vi "Configure C4209.vi"(8 "error in (no error)":errorcluster, 11 "C4209 PNA":refnum<class "C4209 PNA.lvclass">) -> (0 "error out":errorcluster, 3 "C4209 PNA out":refnum<class "C4209 PNA.lvclass">)   [LabVIEW 2017, in "C4209 PNA.lvclass"]
uses:
  C4209 PNA.lvclass
  C4209 PNA.lvclass/C4209 PNA.ctl
  <instrlib>/CMT S2 Series VNA/CMT S2 Series VNA.lvlib
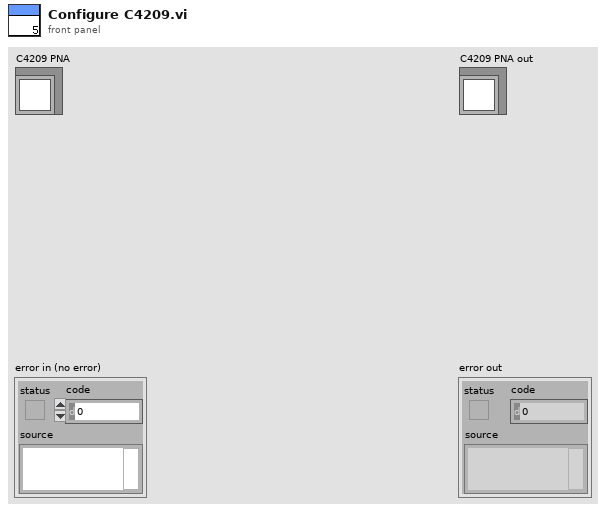
[diagram p1: front panel]
types:
  T1 = typedef "N5222AConfig.ctl" = cluster{"ResourceName":string, "Enable":bool, "Channel":i32, "CalFileName":string, "MeasName":string, "TempDatFile":string, "Power, dBm":dbl, "NumPoints":i32, "Start Freq, Hz":dbl, "Stop Freq, Hz":dbl, "NumAverages":i32, "Sweep Type":i32}
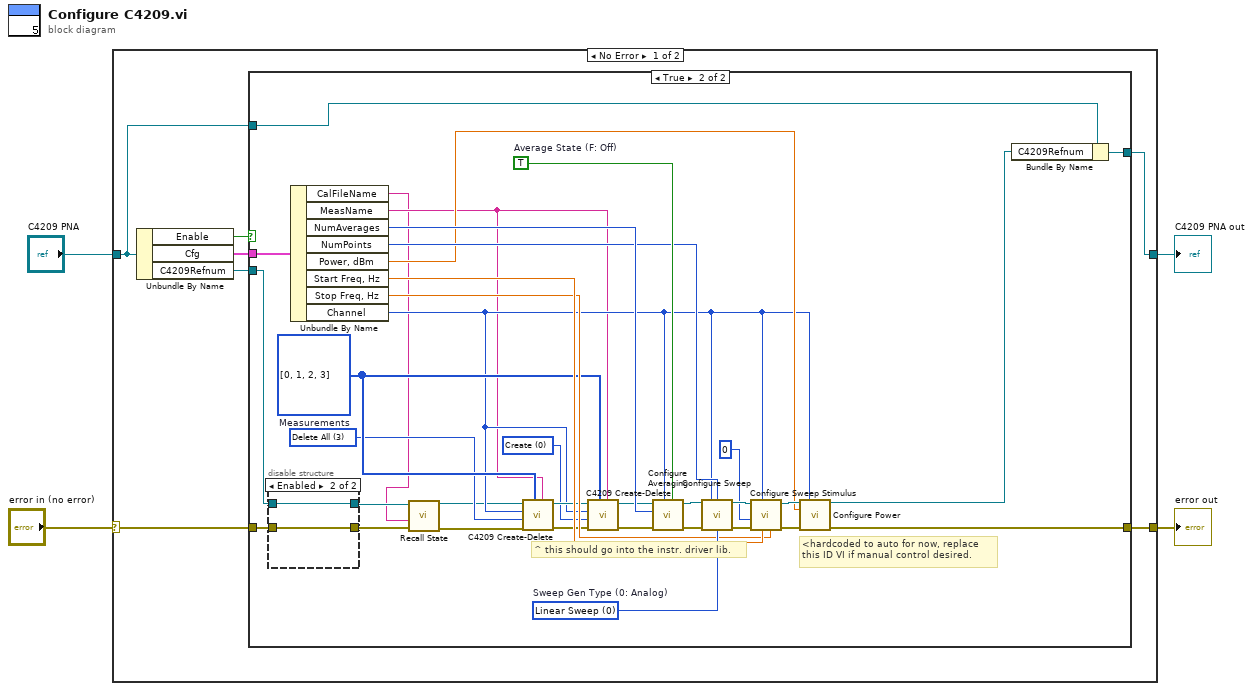
[diagram p0: block diagram]
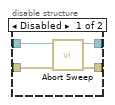
[diagram p3: hidden frame]
diagram:
  n1 = case shown="No Error" "error in (no error)" {
    selector: "error in (no error)" -> [w8 w56]
    tunnel: [w5 w56] -> w3
    tunnel: [w6 w55] -> w1
    tunnel: "C4209 PNA" -> [w7 w55]
    frame No Error {
      n2 = Unbundle By Name(w7) -> ("Enable"=w11:bool, "Cfg"=w10:T1, "C4209Refnum"=w9:refnum<k7>)
      n3 = case shown="True" w11 {
        tunnel: w10 -> [_ w48]
        tunnel: [w12 w31] -> w5
        tunnel: w8 -> [w12 w47]
        tunnel: [w13 w44] -> w6
        tunnel: w7 -> [w13 w45]
        tunnel: w9 -> [_ w46]
        frame False {
        }
        frame True {
          w39 = 0 items=["Linear Sweep", "Logarithmic Sweep", "Segment Sweep", "Power Sweep"]  # Sweep Gen Type (0: Analog)
          w43 = TRUE  # Average State (F: Off)
          w23 = u16 0 items=["Create", "Delete", "Select", "Delete All"] ("Mode (0: Create)")
          w24 = u16 3 items=["Create", "Delete", "Select", "Delete All"] ("Mode (0: Create)")
          w25 = i32[] [0, 1, 2, 3] items=["S11", "S21", "S12", "S22", "A", "B", "R1", "R2", "A/B", "B/A"]  # Measurements
          # "^ this should go into the instr. driver lib."
          # "<hardcoded to auto for now, replace\nthis ID VI if manual control desired."
          n4 = disable-structure shown="Enabled" {
            disable-tunnel: [w50 w53] -> w17
            disable-tunnel: w47 -> [w49 w53]
            disable-tunnel: w46 -> [w52 w54]
            disable-tunnel: [w51 w54] -> w18
            frame Disabled {
              n5 = call <instrlib>:"Abort Sweep.vi"("error in (no error)"=w49, "Reference in"=w52) -> ("error out"=w50:errorcluster, "Reference out"=w51:refnum<k7>)  [unwired: 8 in]
            }
            frame Enabled {
            }
          }
          n6 = Unbundle By Name(w48) -> ("CalFileName"=w14:string, "MeasName"=w21:string, "NumAverages"=w42:i32, "NumPoints"=w38:i32, "Power, dBm"=w28:dbl, "Start Freq, Hz"=w35:dbl, "Stop Freq, Hz"=w34:dbl, "Channel"=w22:i32)
          n7 = call <instrlib>:"Recall State.vi"("error in (no error)"=w17, "File Name ()"=w14, "Reference in"=w18) -> ("error out"=w16:errorcluster, "Reference out"=w15:refnum<k7>)  [unwired: 7 in]
          n8 = call "C4209 Create-Delete.vi"("Reference in"=w15, "Channel (1)"=w22, "Mode (0: Create)"=w24, "error in"=w16, "Measurements"=w25, "Measurement Name"=w21) -> ("Reference out"=w26:refnum<k7>, "Error Out"=w27:errorcluster)  [unwired: 3 in]
          n9 = call "C4209 Create-Delete.vi"("Reference in"=w26, "Channel (1)"=w22, "Mode (0: Create)"=w23, "error in"=w27, "Measurements"=w25, "Measurement Name"=w21) -> ("Reference out"=w20:refnum<k7>, "Error Out"=w19:errorcluster)  [unwired: 3 in]
          n10 = call <instrlib>:"Configure Averaging.vi"("Averaging State (F: Off)"=w43, "Channel (1)"=w22, "error in (no error)"=w19, "Factor (16)"=w42, "Reference in"=w20) -> ("error out"=w41:errorcluster, "Reference out"=w40:refnum<k7>)  [unwired: 5 in]
          n11 = call <instrlib>:"Configure Sweep.vi"("Reference in"=w40, "Channel (1)"=w22, "Number of Measurement Points (201)"=w38, "error in (no error)"=w41, "Sweep Type (0: Linear Sweep)"=w39) -> ("Reference out"=w36:refnum<k7>, "error out"=w37:errorcluster)  [unwired: 9 in]
          n12 = call <instrlib>:"Configure Sweep Stimulus.vi"("Stop/Span"=w34, "Start/Center"=w35, "Channel (1)"=w22, "error in (no error)"=w37, "Stimulus Mode (0: Start/Stop)"=0, "Reference in"=w36) -> ("error out"=w32:errorcluster, "Reference out"=w29:refnum<k7>)  [unwired: 4 in]
          n13 = call <instrlib>:"Configure Power.vi"("Reference in"=w29, "Channel (1)"=w22, "Power Level (0.0)"=w28, "error in (no error)"=w32) -> ("Reference out"=w30:refnum<k7>, "error out"=w31:errorcluster)  [unwired: 10 in]
          n14 = Bundle By Name(cluster=w45, "C4209Refnum"=w30) -> (w44:refnum<class "C4209 PNA.lvclass">)
        }
      }
    }
    frame Error {
    }
  }
  "error out" <- w3
  "C4209 PNA out" <- w1
